vi "Simple SCP File Download.vi"() -> ()   [LabVIEW 2018]
doc: "Downloads, or receives, a relatively small file from a remote SSH server. This is similar to the SCP command line utility when transferring, or copying, a remote file to a local destination. If performance is poor or memory is limited on the local machine, then it could be because the file is relatively large and this implementation is not very efficient for relatively large files."
uses:
  Toolkit/File Info/File Info.lvclass/File Info.ctl
  Toolkit/SSH/SSH.lvclass/SSH.ctl
  Toolkit/SSH/Utility/Read Shared Library.vi
  Toolkit/Session/Support/Create from SSH.vi
  Toolkit/Session/Support/Password Authentication.vi
  Toolkit/File Info/Support/Create from Session.vi
  Toolkit/Channel/Support/Create from SCP Receive.vi
  Toolkit/Support/Check Status.vi
  Toolkit/File Info/Support/Destroy to Channel.vi
  Toolkit/Channel/Support/Destroy to Session.vi
  Toolkit/Session/Support/Destroy to SSH.vi
  Toolkit/SSH/SSH.lvclass
  Toolkit/Session/Session.lvclass
  Toolkit/Channel/Channel.lvclass
  Toolkit/File Info/File Info.lvclass
panel:
  in  "Remote File":string
  in  "Local File":path
  in  "Remote SSH Server":string
  in  "Password":string
  in  "Username":string
  # "Overview: Demonstrates transferring, or downloading, a remote file from a SSH server, similar to the SCP command line utility\nInstructions:\n1. Enter the IP address or host name of the remote SSH server. This can be a CompactRIO (cRIO) running the National Instruments Linux Real-Time (NI Linux RT) operating system with the Enable Secure Shell Server (sshd) checkbox checked. \n2. Enter a username. If using a cRIO with a default configuration, then the username is \"admin\".\n3. Enter a password for the username. If using a cRIO with a default configuration, then the password is blank (empty).\n4. Enter the path and/or filename of the remote file to download. Typically, this is a POSIX/UNIX file path with a backslash, \"/\", use to separate directories and the default directory is the remote user's home directory, i.e. \"/home/admin\" on a default configured cRIO.\n5. Select a destination on the local computer for the transfer/download from the remote SSH server.\n6. Run this VI."
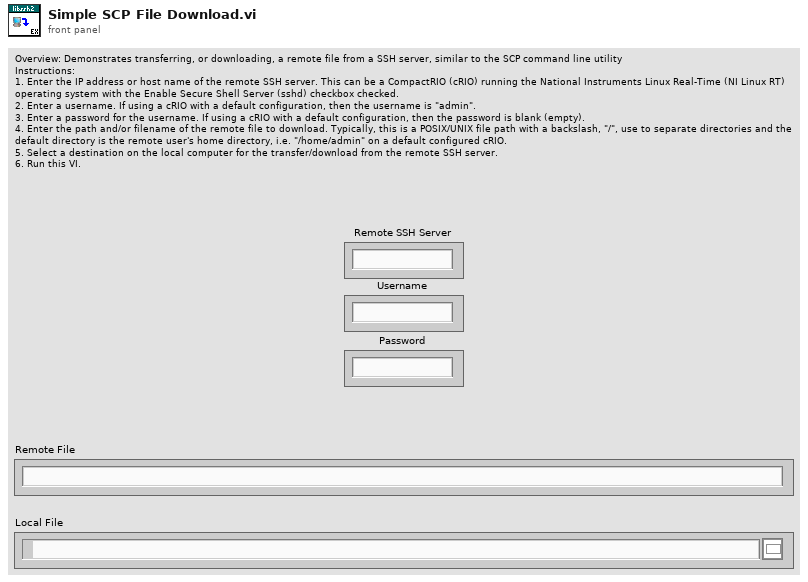
[diagram p1: front panel]
types:
  T1 = enum16{"open", "replace", "create", "open or create", "replace or create", "replace or create with confirmation"}
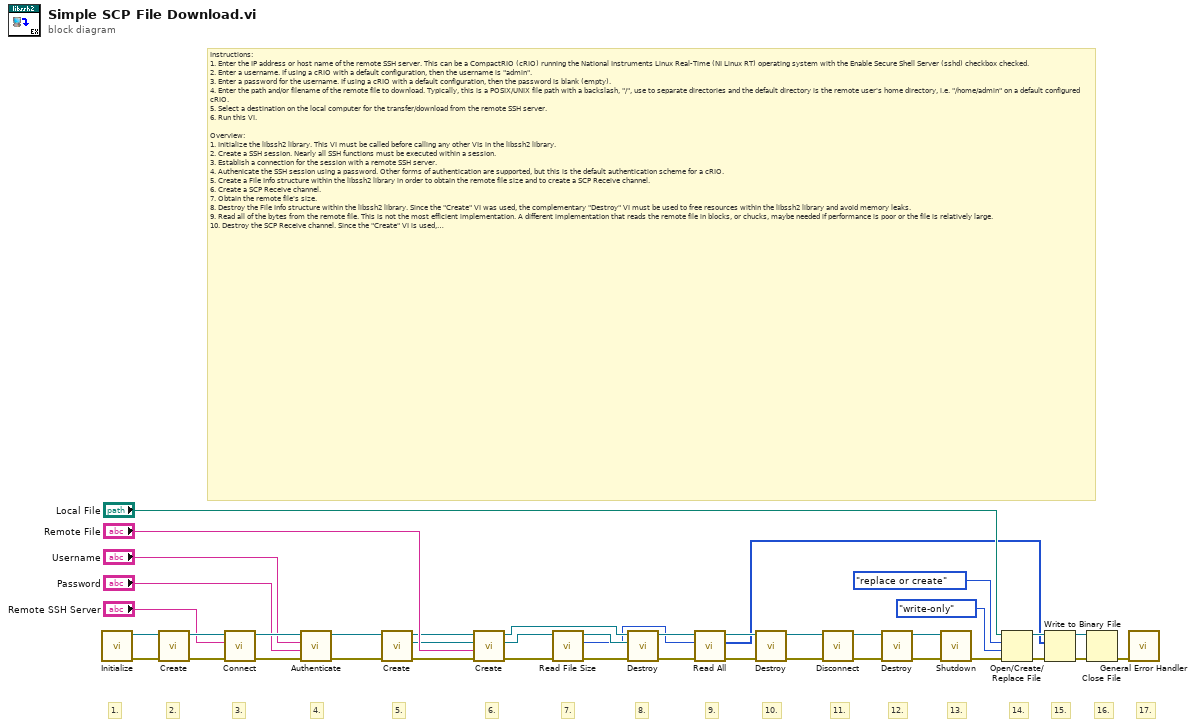
[diagram p0: block diagram]
diagram:
  # "17."
  # "16."
  # "15."
  # "14."
  # "13."
  # "12."
  # "11."
  # "10."
  # "9."
  # "8."
  # "7."
  # "6."
  # "5."
  # "4."
  # "3."
  # "2."
  # "1."
  # "Instructions:\n1. Enter the IP address or host name of the remote SSH server. This can be a CompactRIO (cRIO) running the National Instruments Linux Real-Time (NI Linux RT) operating system with the Enable Secure Shell Server (sshd) checkbox checked. \n2. Enter a username. If using a cRIO with a default configuration, then the username is \"admin\".\n3. Enter a password for the username. If using a cRIO with a default configuration, then the password is blank (empty).\n4. Enter the path and/or filename of the remote file to download. Typically, this is a POSIX/UNIX file path with a backslash, \"/\", use to separate directories and the default directory is the remote user's home directory, i.e. \"/home/admin\" on a default configured cRIO.\n5. Select a destination on the local computer for the transfer/download from the remote SSH server.\n6. Run this VI.\n\nOverview:\n1. Initialize the libssh2 library. This VI must be called before calling any other VIs in the libssh2 library.\n2. Create a SSH session. Nearly all SSH functions must be executed within a session.\n3. Establish a connection for the session with a remote SSH server.\n4. Authenicate the SSH session using a password. Other forms of authentication are supported, but this is the default authentication scheme for a cRIO. \n5. Create a File Info structure within the libssh2 library in order to obtain the remote file size and to create a SCP Receive channel.\n6. Create a SCP Receive channel.\n7. Obtain the remote file's size.\n8. Destroy the File Info structure within the libssh2 library. Since the \"Create\" VI was used, the complementary \"Destroy\" VI must be used to free resources within the libssh2 library and avoid memory leaks.\n9. Read all of the bytes from the remote file. This is not the most efficient implementation. A different implementation that reads the remote file in blocks, or chucks, maybe needed if performance is poor or the file is relatively large.\n10. Destroy the SCP Receive channel. Since the \"Create\" VI is used, the complementary \"Destroy\" VI must be used to free resources within the libssh2 library.\n11. Disconnect from the remote SSH server.\n12. Destroy the session to free resources within the libssh2 library.\n13. Shutdown the libssh2 library. This VI must be last VI called for the libssh2 library. No other libssh2 VIs should be called once this VI is executed.\n14. Create or replace (overwrite) a file to write the read contents from the remote file.\n15. Write the data from the remote file.\n16. Close the file. This is not strictly necessary, but it is good practice.\n17. Provide some error handling and reporting. Libssh2 errors will be in the -8100 range."
  n1 = call "Initialize.vi"() -> ("Error Out"=w27:errorcluster, "SSH"=w26:refnum<class "SSH.lvclass">)  [unwired: 10 in]
  n2 = call-poly "Create.vi"("Error In"=w27, "SSH"=w26) -> ("Error Out"=w40:errorcluster, "Sesssion"=w41:refnum<class "Session.lvclass">)  [unwired: 8 in]
  n3 = call "Connect.vi"("Error In"=w40, "Address"="Remote SSH Server", "Session In"=w41) -> ("Error Out"=w38:errorcluster, "Sesssion Out"=w39:refnum<class "Session.lvclass">)  [unwired: 7 in]
  n4 = call-poly "Authenticate.vi"("Error In"=w38, "Password"="Password", "Username"="Username", "Session In"=w39) -> ("Error Out"=w22:errorcluster, "Sesssion Out"=w25:refnum<class "Session.lvclass">)  [unwired: 6 in]
  n5 = call-poly "Create.vi"("Error In"=w22, "Session In"=w25) -> ("Error Out"=w21:errorcluster, "File Info"=w23:refnum<class "File Info.lvclass">, "Session Out"=w24:refnum<class "Session.lvclass">)  [unwired: 7 in]
  n6 = call-poly "Create.vi"("Error In"=w21, "Remote Source Path"="Remote File", "File Info In"=w23, "Session"=w24) -> ("Error Out"=w18:errorcluster, "File Info Out"=w19:refnum<class "File Info.lvclass">, "Channel"=w20:refnum<class "Channel.lvclass">)  [unwired: 5 in]
  n7 = call "Read File Size.vi"("Error In"=w18, "File Info In"=w19) -> ("Error Out"=w16:errorcluster, "File Size"=w4:u64, "File Info Out"=w17:refnum<class "File Info.lvclass">)  [unwired: 7 in]
  n8 = call-poly "Destroy.vi"("Error In"=w16, "File Info"=w17, "Channel In"=w20) -> ("Error Out"=w5:errorcluster, "Channel Out"=w6:refnum<class "Channel.lvclass">)  [unwired: 7 in]
  n9 = call "Read All.vi"("Error In"=w5, "Total Read Size"=w4, "Channel In"=w6) -> ("Error Out"=w3:errorcluster, "Data"=w1:u8[], "Channel Out"=w2:refnum<class "Channel.lvclass">)  [unwired: 6 in]
  n10 = call-poly "Destroy.vi"("Error In"=w3, "Channel"=w2) -> ("Error Out"=w33:errorcluster, "Session"=w34:refnum<class "Session.lvclass">)  [unwired: 8 in]
  n11 = call "Disconnect.vi"("Error In"=w33, "Session In"=w34) -> ("Error Out"=w31:errorcluster, "Sesssion Out"=w32:refnum<class "Session.lvclass">)  [unwired: 8 in]
  n12 = call-poly "Destroy.vi"("Error In"=w31, "Session"=w32) -> ("Error Out"=w29:errorcluster, "SSH"=w30:refnum<class "SSH.lvclass">)  [unwired: 8 in]
  n13 = call "Shutdown.vi"("Error In"=w29, "SSH"=w30) -> ("Error Out"=w15:errorcluster)  [unwired: 9 in]
  n14 = Open/Create/Replace File(file path (use dialog)="Local File", error in=w15, operation (0:open)=T1."replace or create", access (0:read/write)=enum16{"read/write", "read-only", "write-only"}."write-only") -> (refnum out=w11:refnum<file>, error out=w10:errorcluster)  [unwired: 2 in, 1 out]
  n15 = Write to Binary File(file (use dialog)=w11, data=w1, error in=w10) -> (refnum out=w9:refnum<file>, error out=w8:errorcluster)  [unwired: 3 in, 1 out]
  n16 = Close File(refnum=w9, error in=w8) -> (error out=w7:errorcluster)  [unwired: 1 out]
  n17 = call <vilib>:"General Error Handler.vi"("error in (no error)"=w7) -> ()  [unwired: 10 in, 5 out]
